vi "Target.vi"   [LabVIEW 2025]
uses:
  <vilib>/eio/utilities/niEioResolveVilibRelativePath.vi
  <vilib>/rvi/interface/RandomDataEmulation/niFpgaRandomDataHandleErrors.vi
  <vilib>/rvi/DataTransferAndStorage/Container/XNode/niFpgaContainer.xnode
  <vilib>/rvi/interface/RandomDataEmulation/nirviRandomDataFpgaReadWriteTemplate.vi
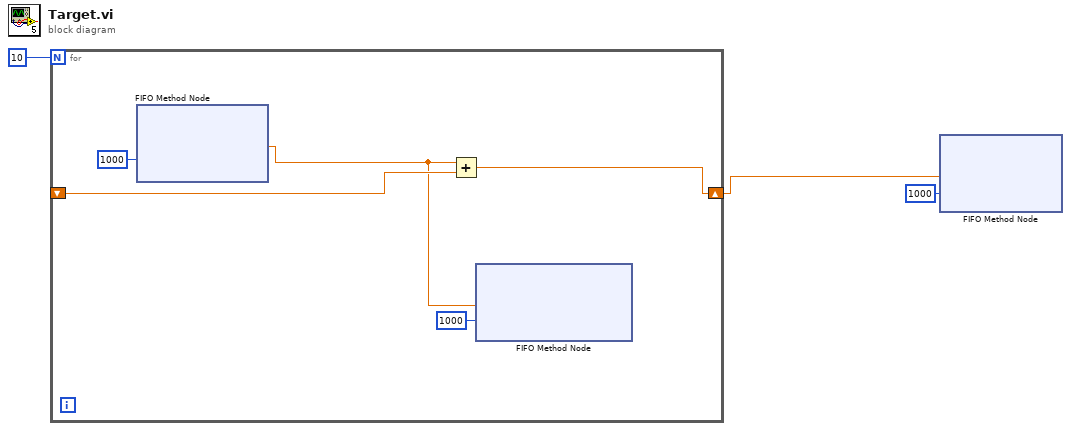
[diagram p0: block diagram]
diagram:
  n1 = for {
    N: 10 -> [_]
    shift-right: [w7] -> w1
    shift-left: _ -> [w6]
    n2 = xnode ("FIFO Method Node")("Timeout"=1000) -> ("Element"=w5:sgl)  [unwired: 1 in, 2 out]
    n3 = Add(x=w5, y=w6) -> (x+y=w7:sgl)
    n4 = xnode ("FIFO Method Node")("Element"=w5, "Timeout"=1000) -> ()  [unwired: 1 in, 2 out]
  }
  n5 = xnode ("FIFO Method Node")("Element"=w1, "Timeout"=1000) -> ()  [unwired: 1 in, 2 out]
